vi "Cholesky Factorization Rank-1 Update (DBL).vi"(9 "method":i32(ring) items=["Update", "Downdate"], 10 "X":dbl[](array[numeric]), 11 "R":T1) -> (0 "error":i32, 3 "Updated R":T1)   [LabVIEW 2020, in "NI_AAL_LinAlg.lvlib"]
doc: "Performs Cholesky factorization on the rank-1 updated Cholesky matrix. The VI performs Cholesky factorization directly on the known factored matrix instead of the updated matrix."
uses:
  <vilib>/Analysis/NI_AAL_LinAlg.lvlib
  <vilib>/Analysis/Matrix/Datatypes/RealMatrix.ctl
  <vilib>/Analysis/Matrix/NI_Matrix.lvlib
panel:
  # "Cholesky Factorization Rank-1 Update (DBL)"
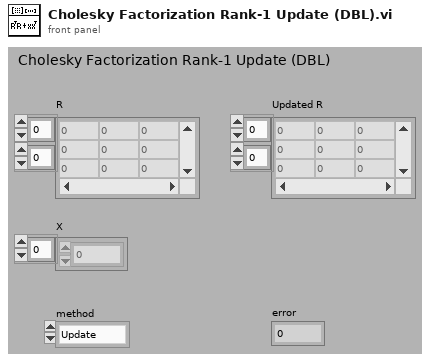
[diagram p1: front panel]
types:
  T1 = typedef "NI_Matrix.lvlib/RealMatrix.ctl" = dbl[][]
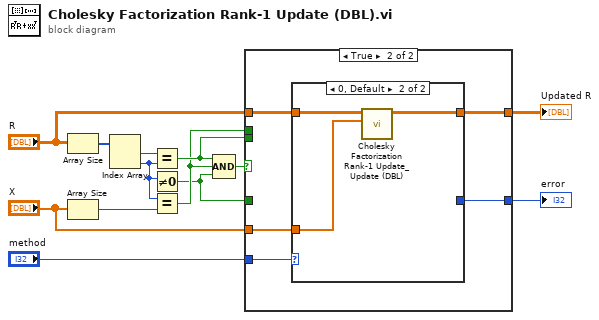
[diagram p0: block diagram]
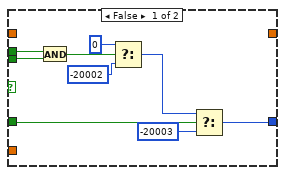
[diagram p2: hidden frame]
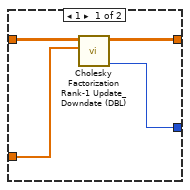
[diagram p3: hidden frame]
diagram:
  n1 = Array Size(array="R") -> (size(s)=w13:i32[])
  n2 = Array Size(array="X") -> (size(s)=w12:i32)
  n3 = Index Array(array=w13) -> (element #1=w9:i32, element #2=w10:i32)  [unwired: 2 in]
  n4 = Equal?(x=w9, y=w10) -> (x = y?=w3:bool)
  n5 = Not Equal To 0?(x=w10) -> (x != 0?=w1:bool)
  n6 = Equal?(x=w10, y=w12) -> (x = y?=w2:bool)
  n7 = Compound Arithmetic op=AND(w3, w2, w1) -> (w8:bool)
  n8 = case shown="True" w8 {
    tunnel: [_ w27] -> w5
    tunnel: "X" -> [_ w25]
    tunnel: "R" -> [_ w26]
    tunnel: [w14 w23] -> w11
    tunnel: "method" -> [_ w24]
    tunnel: w1 -> [w22 _]
    tunnel: w3 -> [w19 _]
    tunnel: w2 -> [w20 _]
    frame False {
      n9 = And(x=w20, y=w19) -> (x .and. y?=w16:bool)
      n10 = Select(t=0, s=w16, f=-20002 ("t")) -> (s? t:f=w15:i32)
      n11 = Select(t=w15, s=w22, f=-20003) -> (s? t:f=w14:i32)
    }
    frame True {
      n12 = case shown="0, Default" w24 {
        tunnel: w26 -> [w30 w34]
        tunnel: w25 -> [w28 w32]
        tunnel: [w31 w33] -> w27
        tunnel: [w29 _] -> w23
        frame 1 {
          n13 = call <vilib>:"Cholesky Factorization Rank-1 Update_Downdate (DBL).vi"("X"=w28, "R"=w30) -> ("error"=w29:i32, "Updated R"=w31:T1)  [unwired: 8 in]
        }
        frame 0, Default {
          n14 = call <vilib>:"Cholesky Factorization Rank-1 Update_Update (DBL).vi"("X"=w32, "R"=w34) -> ("Updated R"=w33:T1)  [unwired: 9 in]
        }
      }
    }
  }
  "error" <- w11
  "Updated R" <- w5
